vi "Autonomous Independent - Copy.vi"   [LabVIEW 2016]
doc: "This VI is called when autonomous begins, and will automatically be terminated when autonomous ends. You can carry out timed or sensor driven robot movement independently without needing to return to the caller."
uses:
  <userlib>/836-libraries/Drive/Drive_Code/Drive_Code_Support/Sensor_Cluster.ctl
  <userlib>/836-libraries/Drive/Drive_Code/Drive_Code_Support/Camera_Cluster.ctl
  <userlib>/836-libraries/Drive/Drive_Code/Drive_Code_Support/Drive_Code_Notifier.ctl
  <userlib>/836-libraries/Drive/Drive_Code/Drive_Code_Support/Drive_Code_Command.ctl
  <userlib>/836-libraries/Drive/Drive_Code/Logging_Data.ctl
  <userlib>/836-libraries/Drive/Drive_Code/Drive_Code_Support/Drive_Code_PID_Bundle.ctl
  <userlib>/836-libraries/Drive/Drive_Code/Drive_Code_Support/Drive_Loop_Cheesey_Drive.vi
panel:
  # "Be sure to right-click and choose Data Operations>>Make Current Value default if you want to save the array values with the VI"
  # "(73)"
  # "(64)"
  # "(48)"
  # "(76)"
  # "(64)"
  # "0.8"
  # "0.5 Right"
types:
  T1 = typedef "Sensor_Cluster.ctl" = cluster{"Gyro Data":cluster{"Gyro RT FIFO":refnum<k33>, "Gyro Current":dbl, "Gyro Hold":dbl}, "Encoder Data":cluster{"Encoder RT FIFO":refnum<k33>, "Encoder Current":dbl, "Encoder Hold":dbl}, "Camera Data":cluster{"Camera RT FIFO":refnum<k33>, "Camera Current":T2}}
  T2 = typedef "Camera_Cluster.ctl" = cluster{" Angle":dbl, "Valid":bool}
  T3 = cluster{"Cluster":T1, "Drive Command rt fifo":refnum<k33>, "Logging Data":refnum<k33>, "PID Update":refnum<notifier>}
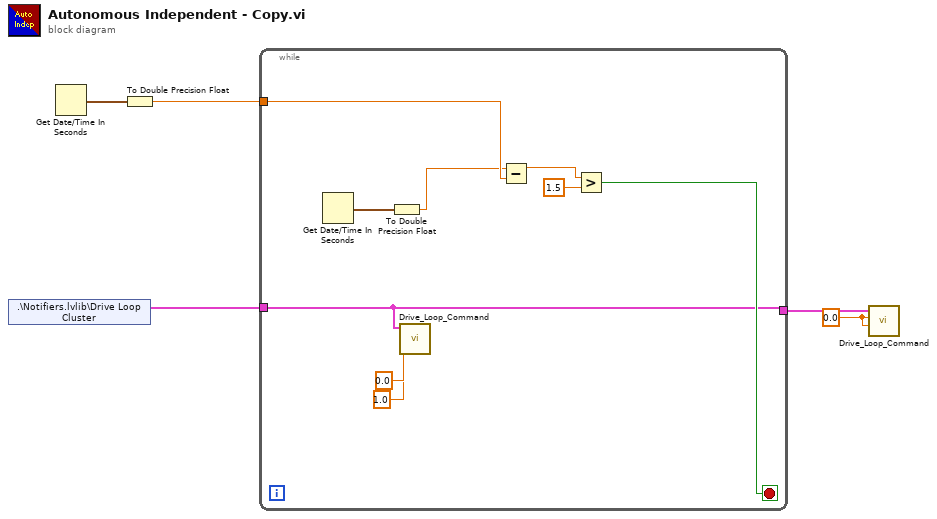
[diagram p0: block diagram]
diagram:
  w1 = 0.0 ("Throttle")
  n1 = shared-variable ".\\Notifiers.lvlib\\Drive Loop Cluster"() -> (w3:T3)  [unwired: 1 in, 1 out]
  n2 = Get Date/Time In Seconds() -> (seconds since 1Jan1904=w5:timestamp)
  n3 = To Double Precision Float(number=w5) -> (double precision float=w4:dbl)
  n4 = while {
    tunnel: w4 -> [w13]
    tunnel: w3 -> [w6]
    tunnel: [w6] -> w2
    stop <- w7 stop-if-true
    n5 = Get Date/Time In Seconds() -> (seconds since 1Jan1904=w14:timestamp)
    n6 = To Double Precision Float(number=w14) -> (double precision float=w12:dbl)
    n7 = call-poly <userlib>:"Drive_Loop_Command.vi"("Wheel"=0.0, "Throttle"=1.0, "Drive Loop Cluster"=w6) -> ()  [unwired: 9 in]
    n8 = Subtract(x=w12, y=w13) -> (x-y=w11:dbl)
    n9 = Greater?(x=w11, y=1.5) -> (0:w7:bool)
  }
  n10 = call-poly <userlib>:"Drive_Loop_Command.vi"("Wheel"=w1, "Throttle"=w1, "Drive Loop Cluster"=w2) -> ()  [unwired: 9 in]
